vi "get_status_error.vi"(8 "error in (no error)":errorcluster, 11 "LightSourceMH110125Tsunami in":refnum<class "LightSourceMH110125Tsunami.lvclass">) -> (0 "error out":errorcluster, 3 "LightSourceMH110125Tsunami out":refnum<class "LightSourceMH110125Tsunami.lvclass">)   [LabVIEW 2010, in "LightSourceMH110125Tsunami.lvclass"]
uses:
  LightSourceMH110125Tsunami.lvclass
  LightSourceScaffold/LightSourceScaffold/LightSourceScaffold.lvclass
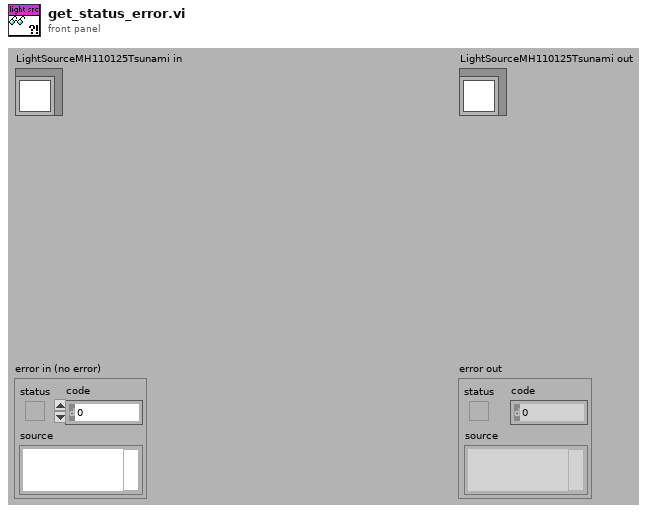
[diagram p1: front panel]
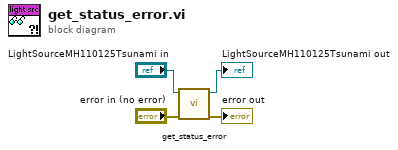
[diagram p0: block diagram]
diagram:
  n1 = call-parent "get_status_error.vi"("error in (no error)"="error in (no error)", "LightSourceScaffold in"="LightSourceMH110125Tsunami in") -> ("error out"=→"error out":errorcluster, "LightSourceScaffold out"=→"LightSourceMH110125Tsunami out":refnum<class "LightSourceMH110125Tsunami.lvclass">)  [unwired: 8 in]
